vi "Z Aux Direct Get Merge.vi"(8 "error in (no error)":errorcluster caption="错误输入（无错误）", 9 "piValue":i32, 10 "iaxis":i32, 11 "handle":u32) -> (0 "error out":errorcluster caption="错误输出", 1 "piValue out":i32, 2 "function return":i32, 3 "handle out":u32)   [LabVIEW 2015, in "zauxdll.lvlib"]
doc: "int32 __stdcall ZAux_Direct_GetMerge(ZMC_HANDLE handle, int iaxis, int *piValue);"
uses:
  zauxdll.lvlib
  zauxdll.dll
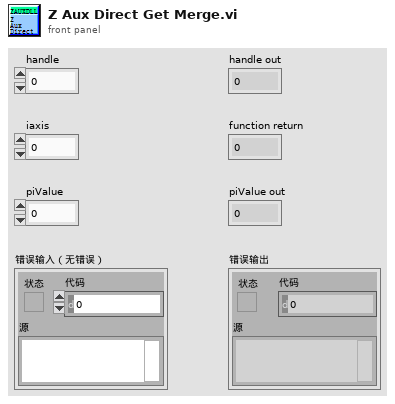
[diagram p1: front panel]
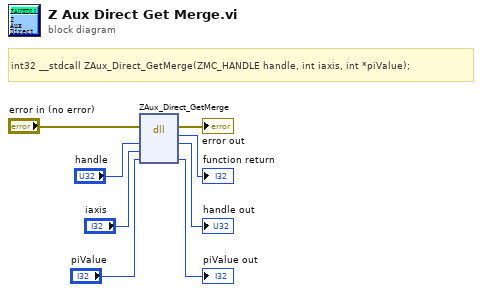
[diagram p0: block diagram]
diagram:
  # "int32 __stdcall ZAux_Direct_GetMerge(ZMC_HANDLE handle, int iaxis, int *piValue);"
  n1 = dll-call lib="C:/Users/VIC/Desktop/GOGORO_Oringnal - Panasonic/system/LLB/zmotion/zaux/zauxdll.*" fn="ZAux_Direct_GetMerge"(error in="error in (no error)", "handle"="handle", "iaxis"="iaxis", "piValue"="piValue") -> (error out=→"error out":errorcluster, →"function return":i32, "handle"=→"handle out":u32, "piValue"=→"piValue out":i32)  [unwired: 3 in, 1 out]
